vi "ConfigMeas.vi"(0 "reference in":refnum<class "LCR_BK891.lvclass">, 5 "Function (4: Cp-D)":u16(ring)=4 items=["Cs-Q", "Cs-D", "Cs-R", "Cp-Q", "Cp-D", "Cp-R", "Cp-G", "Ls-Q", "Ls-D", "Ls-R", "Lp-Q", "Lp-D", "Lp-R", "Lp-G", "Z-th", "Y-th", "R-X", "G-B", "DCR"], 7 "Range (1:Auto)":u16(ring)=1 items=["Hold", "Auto"], 9 "Meas_Speed":enum16{"Slow", "Fast"}(ring)=enum."Fast", 11 "error in (no error)":errorcluster) -> (4 "reference in":refnum<class "LCR_BK891.lvclass">, 15 "error out":errorcluster)   [LabVIEW 2022 SP3, in "LCR_BK891.lvlib" / "LCR_BK891.lvclass"]
uses:
  LCR_BK891.lvclass
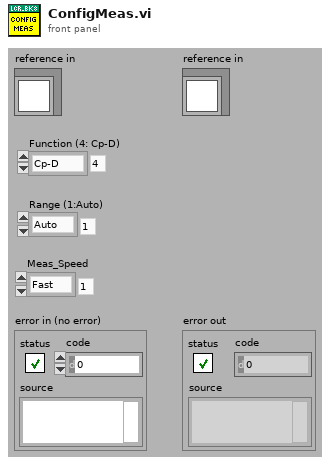
[diagram p1: front panel]
types:
  T1 = typedef "LCR_BK891.lvlib/LCR_BK891.lvclass/ObjectAttributes.ctl" = cluster{"Config":T2, "VISA Ref":refnum<visa-resource-name>, "Function":u16, "Range":u16, "Measurement Speed":u16, "Signal Frequency":dbl, "Signal Level":u8, "Measured Primary Reading":dbl, "Measured Secondary Reading":dbl}
  T2 = typedef "LCR_BK891.lvlib/LCR_BK891.lvclass/Config.ctl" = cluster{"VISA":refnum<visa-resource-name>}
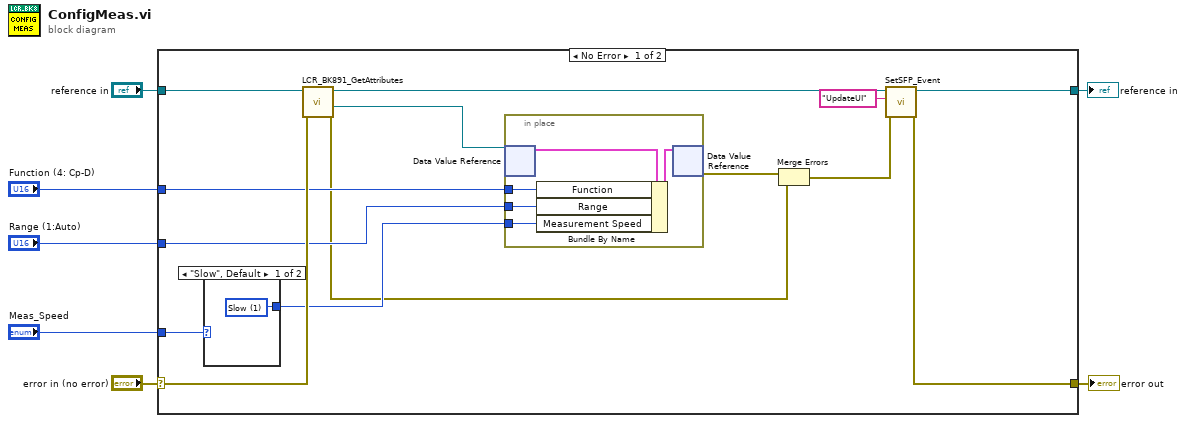
[diagram p0: block diagram]
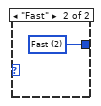
[diagram p2: hidden frame]
diagram:
  n1 = case shown="No Error" "error in (no error)" {
    selector: "error in (no error)" -> [w21 w30]
    tunnel: [w14 w30] -> w6
    tunnel: [w15 w29] -> w4
    tunnel: "reference in" -> [w20 w29]
    tunnel: "Range (1:Auto)" -> [w17 _]
    tunnel: "Function (4: Cp-D)" -> [w18 _]
    tunnel: "Meas_Speed" -> [w10 _]
    frame No Error {
      n2 = case shown="\"Slow\", Default" w10 {
        tunnel: [w22 w23] -> w9
        frame "Slow", Default {
          w22 = u16 1 items=["Slow"=1, "Fast"=2] ("Measurement Speed (2:Fast)")
        }
        frame "Fast" {
          w23 = u16 2 items=["Slow"=1, "Fast"=2] ("Measurement Speed (2:Fast)")
        }
      }
      n3 = call "LCR_BK891_GetAttributes.vi"("error in (no error)"=w21, "reference in"=w20) -> ("error out"=w8:errorcluster, "DataRef"=w19:refnum<data-value>, "reference out"=w16:refnum<class "LCR_BK891.lvclass">)  [unwired: 6 in, 1 out]
      n4 = in-place {
        in-place-border: w18 -> [w26]
        in-place-border: w17 -> [w25]
        in-place-border: w9 -> [w24]
        n5 = in-place-dvr #1(w19) -> (w28:T1)  [unwired: 1 out]
        n6 = Bundle By Name(cluster=w28, "Function"=w26, "Range"=w25, "Measurement Speed"=w24) -> (w27:T1)
        n7 = in-place-dvr #1(w27) -> (w13:errorcluster)  [unwired: 1 out]
      }
      n8 = Merge Errors(w13, w8) -> (w12:errorcluster)
      n9 = call-dynamic "SetSFP_Event.vi"("error in (no error)"=w12, "msg"="UpdateUI", "reference in"=w16) -> ("error out"=w14:errorcluster, "reference out"=w15:refnum<class "LCR_BK891.lvclass">)  [unwired: 7 in]
    }
    frame Error {
    }
  }
  "error out" <- w6
  "reference in" <- w4
